vi "Fetch Multi Eval Meas ACLR Detected Allocation Results.vi"(8 "error in (no error)":errorcluster, 10 "Instance (1)":T2=1, 11 "VISA resource name":refnum<visa-resource-name>) -> (0 "error out":errorcluster, 1 "Detected Allocation":T1, 2 "Reliability":i32, 3 "VISA resource name out":refnum<visa-resource-name>)   [LabVIEW 2015, in "Rohde&Schwarz CMXP NR FR2 Measurement.lvlib"]
doc: "Returns the multi eval measurement ACLR results.\n\nAttribute:\nRSCMXPNRFR2M_ATTR_FETCH_MULTI_EVAL_MEASUREMENT_ACLR_DETECTED_ALLOCATION\n\nRemote-control command:\nFETCh:NRMMw:MEAS<i>:MEValuation:ACLR:DALLocation?"
uses:
  <instrlib>/Rohde&Schwarz CMXP NR FR2 Measurement/Rohde&Schwarz CMXP NR FR2 Measurement.lvlib
  <instrlib>/Rohde&Schwarz CMXP NR FR2 Measurement/Private/_Instance.ctl
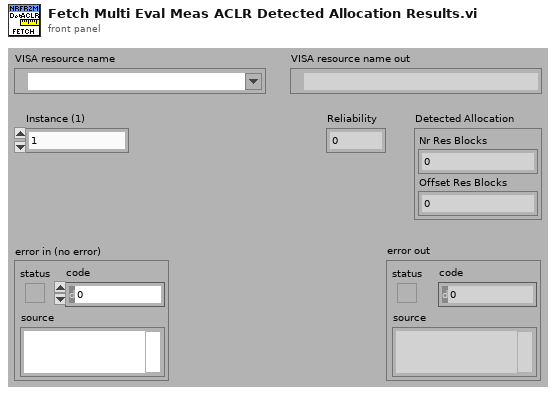
[diagram p1: front panel]
types:
  T1 = cluster{"Nr Res Blocks":i32, "Offset Res Blocks":i32}
  T2 = typedef "Rohde&Schwarz CMXP NR FR2 Measurement.lvlib/_Instance.ctl" = i32
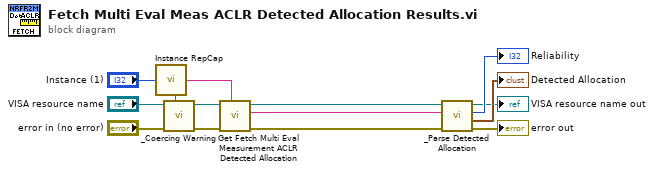
[diagram p0: block diagram]
diagram:
  n1 = call <instrlib>:"Instance RepCap.vi"("Instance In"="Instance (1)") -> ("In Range?"=w4:bool, "RepCap Identifier Out"=w11:string)  [unwired: 1 in]
  n2 = call <instrlib>:"_Coercing Warning.vi"("In Range?"=w4, "error in (no error)"="error in (no error)", "VISA resource name"="VISA resource name") -> ("error out"=w2:errorcluster, "VISA resource name out"=w3:refnum<visa-resource-name>)  [unwired: 7 in]
  n3 = call "Get Fetch Multi Eval Measurement ACLR Detected Allocation"("Repeated Capabilities"=w11, "error in (no error)"=w2, "instrument handle"=w3) -> ("error out"=w10:errorcluster, "Fetch Multi Eval Measurement ACLR Detected Allocation"=w14:string, "instrument handle out"=w9:refnum<visa-resource-name>)  [unwired: 6 in]
  n4 = call <instrlib>:"_Parse Detected Allocation.vi"("error in (no error)"=w10, "Input String"=w14, "VISA resource name"=w9) -> ("error out"=→"error out":errorcluster, "Detected Allocation"=→"Detected Allocation":T1, "Reliability"=→"Reliability":i32, "VISA resource name out"=→"VISA resource name out":refnum<visa-resource-name>)  [unwired: 5 in]
